vi "Get GUID Controls on Constants VI.vi"(8 "error in":errorcluster, 11 "VI in":refnum<vi>) -> (0 "error out":errorcluster, 2 "GUID controls":refnum<vi>[](array[refnum]), 3 "VI out":refnum<vi>)   [LabVIEW 2020, in "Utility.lvlib"]
uses:
  Utility.lvlib
  <vilib>/Utility/traverseref.llb/VI Scripting - Traverse.lvlib
  <vilib>/Utility/traverseref.llb/TRef TravTarget.ctl
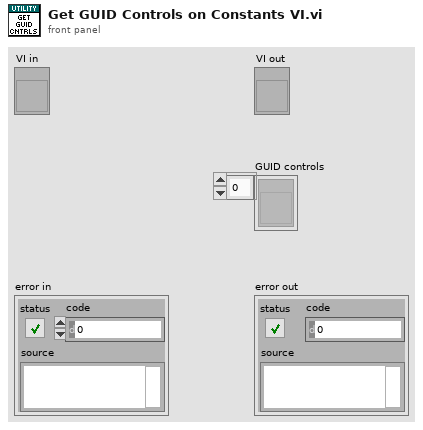
[diagram p1: front panel]
types:
  T1 = typedef "TRef TravTarget.ctl" = enum16{"FP", "BD", "Other"}
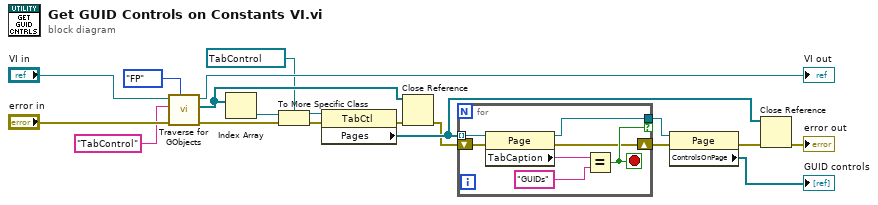
[diagram p0: block diagram]
diagram:
  n1 = call <vilib>:"Traverse for GObjects.vi"("Traverse Target"=TRef_TravTarget."FP", "error in (no error)"="error in", "Class Name"="TabControl", "VI Refnum"="VI in") -> ("error out"=w5:errorcluster, "References"=w6:refnum<vi>[], "dup VI Refnum"=→"VI out":refnum<vi>)  [unwired: 4 in, 1 out]
  n2 = Index Array(array=w6) -> (element=w2:refnum<vi>)  [unwired: 1 in]
  n3 = To More Specific Class(target class=refnum<vi> refnum ("reference"), reference=w2, error in=w5) -> (specific class reference=w1:refnum<vi>, error out=w4:errorcluster)
  n4 = property class="TabCtl"(reference=w1, error in=w4) -> (error out=w13:errorcluster, "Pages"=w18:refnum<vi>[])  [unwired: 1 out]
  n5 = Close Reference(reference=w6, error in (no error)=w13) -> (error out=w16:errorcluster)
  n6 = for {
    tunnel: w18 -> [w26] mode=indexing
    tunnel: [w25] -> w12 if=w24
    shift-right: [w22] -> w14
    shift-left: w16 -> [w23]
    stop <- w24 stop-if-true
    n7 = property class="Page"(reference=w26, error in=w23) -> (reference out=w25:refnum<vi>, error out=w22:errorcluster, "TabCaption"=w20:string)
    n8 = Equal?(x=w20, y="GUIDs") -> (x = y?=w24:bool)
  }
  n9 = property class="Page"(reference=w12, error in=w14) -> (error out=w15:errorcluster, "ControlsOnPage"=→"GUID controls":refnum<vi>[])  [unwired: 1 out]
  n10 = Close Reference(reference=w18, error in (no error)=w15) -> (error out=→"error out":errorcluster)
